vi "Trigger_Coincidence_Logic.vi"(6 "Peak_ch6":u16, 7 "Peak_ch1":u16, 8 "Peak_ch5":u16, 9 "Peak_ch4":u16, 10 "Peak_ch3":u16, 11 "Peak_ch2":u16) -> (3 "Filter-out":bool)   [LabVIEW 2019]
uses:
  SiPM_Tests_Global_Var.vi
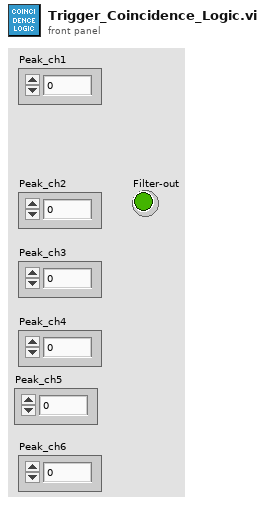
[diagram p1: front panel]
types:
  T1 = enum16{"Coincidence", "Anti-Coincidence", "Don't Care"}
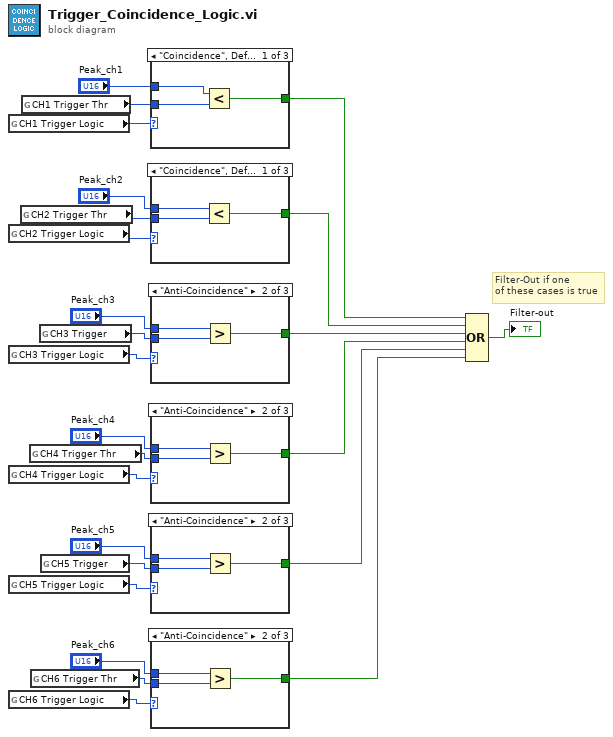
[diagram p0: block diagram]
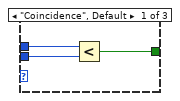
[diagram p2: hidden frame]
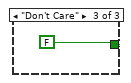
[diagram p3: hidden frame]
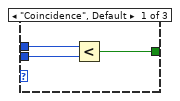
[diagram p4: hidden frame]
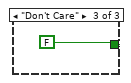
[diagram p5: hidden frame]
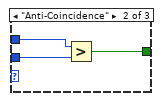
[diagram p6: hidden frame]
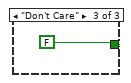
[diagram p7: hidden frame]
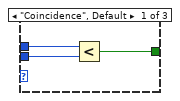
[diagram p8: hidden frame]
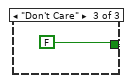
[diagram p9: hidden frame]
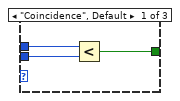
[diagram p10: hidden frame]
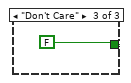
[diagram p11: hidden frame]
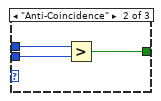
[diagram p12: hidden frame]
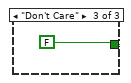
[diagram p13: hidden frame]
diagram:
  # "Filter-Out if one \nof these cases is true"
  n1 = global read "SiPM_Tests_Global_Var.vi" "CH1 Trigger Logic"() -> (w12:T1)
  n2 = global read "SiPM_Tests_Global_Var.vi" "CH2 Trigger Logic"() -> (w13:T1)
  n3 = global read "SiPM_Tests_Global_Var.vi" "CH3 Trigger Logic"() -> (w17:T1)
  n4 = global read "SiPM_Tests_Global_Var.vi" "CH4 Trigger Logic"() -> (w20:T1)
  n5 = global read "SiPM_Tests_Global_Var.vi" "CH5 Trigger Logic"() -> (w7:T1)
  n6 = global read "SiPM_Tests_Global_Var.vi" "CH6 Trigger Logic"() -> (w3:T1)
  n7 = global read "SiPM_Tests_Global_Var.vi" "CH2 Trigger Thr"() -> (w14:u16)
  n8 = global read "SiPM_Tests_Global_Var.vi" "CH1 Trigger Thr"() -> (w11:u16)
  n9 = global read "SiPM_Tests_Global_Var.vi" "CH4 Trigger Thr"() -> (w21:u16)
  n10 = global read "SiPM_Tests_Global_Var.vi" "CH6 Trigger Thr"() -> (w4:u16)
  n11 = global read "SiPM_Tests_Global_Var.vi" "CH3 Trigger"() -> (w16:u16)
  n12 = global read "SiPM_Tests_Global_Var.vi" "CH5 Trigger"() -> (w8:u16)
  n13 = case shown="\"Coincidence\", Default" w12 {
    tunnel: [w28 w31 FALSE] -> w9
    tunnel: w11 -> [w27 w30 _]
    tunnel: "Peak_ch1" -> [w26 w29 _]
    frame "Coincidence", Default {
      n14 = Less?(x=w26, y=w27) -> (x < y?=w28:bool)
    }
    frame "Anti-Coincidence" {
      n15 = Greater?(x=w29, y=w30) -> (0:w31:bool)
    }
    frame "Don't Care" {
    }
  }
  n16 = case shown="\"Coincidence\", Default" w13 {
    tunnel: [w33 w36 FALSE] -> w22
    tunnel: w14 -> [w35 w37 _]
    tunnel: "Peak_ch2" -> [w34 w38 _]
    frame "Coincidence", Default {
      n17 = Less?(x=w34, y=w35) -> (x < y?=w33:bool)
    }
    frame "Anti-Coincidence" {
      n18 = Greater?(x=w38, y=w37) -> (0:w36:bool)
    }
    frame "Don't Care" {
    }
  }
  n19 = case shown="\"Anti-Coincidence\"" w17 {
    tunnel: [w40 w43 FALSE] -> w23
    tunnel: w16 -> [w42 w44 _]
    tunnel: "Peak_ch3" -> [w41 w45 _]
    frame "Coincidence", Default {
      n20 = Less?(x=w41, y=w42) -> (x < y?=w40:bool)
    }
    frame "Anti-Coincidence" {
      n21 = Greater?(x=w45, y=w44) -> (0:w43:bool)
    }
    frame "Don't Care" {
    }
  }
  n22 = case shown="\"Anti-Coincidence\"" w20 {
    tunnel: [w47 w50 FALSE] -> w24
    tunnel: w21 -> [w49 w51 _]
    tunnel: "Peak_ch4" -> [w48 w52 _]
    frame "Coincidence", Default {
      n23 = Less?(x=w48, y=w49) -> (x < y?=w47:bool)
    }
    frame "Anti-Coincidence" {
      n24 = Greater?(x=w52, y=w51) -> (0:w50:bool)
    }
    frame "Don't Care" {
    }
  }
  n25 = case shown="\"Anti-Coincidence\"" w7 {
    tunnel: [w54 w57 FALSE] -> w5
    tunnel: w8 -> [w56 w58 _]
    tunnel: "Peak_ch5" -> [w55 w59 _]
    frame "Coincidence", Default {
      n26 = Less?(x=w55, y=w56) -> (x < y?=w54:bool)
    }
    frame "Anti-Coincidence" {
      n27 = Greater?(x=w59, y=w58) -> (0:w57:bool)
    }
    frame "Don't Care" {
    }
  }
  n28 = case shown="\"Anti-Coincidence\"" w3 {
    tunnel: [w61 w64 FALSE] -> w1
    tunnel: w4 -> [w63 w65 _]
    tunnel: "Peak_ch6" -> [w62 w66 _]
    frame "Coincidence", Default {
      n29 = Less?(x=w62, y=w63) -> (x < y?=w61:bool)
    }
    frame "Anti-Coincidence" {
      n30 = Greater?(x=w66, y=w65) -> (0:w64:bool)
    }
    frame "Don't Care" {
    }
  }
  n31 = Compound Arithmetic op=OR(w9, w22, w23, w24, w5, w1) -> (→"Filter-out":bool)
